vi "contador_logger_global.vi"() -> ()   [LabVIEW 2017]
panel:
  in  "log_count":u64
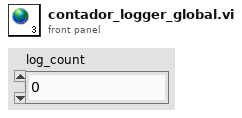
[diagram p1: front panel]
diagram:
